vi "Configuration writer.vi"(0 "Path":T1, 1 "Width (px)":i32=240, 2 "error in (no error)":errorcluster, 3 "Precision (%)":dbl=1.0 min=1.0 max=100.0 step=1.0 format="%#_3g", 4 "Heigth (px)":i32=240, 5 "X offset":i32=693 step=1, 6 "X travel":dbl min=0.0 max=50.0 step=0.0001, 7 "Y offset":i32=406 step=1, 10 "Speed (µm/s)":i32=1000, 11 "Height  step \ndivider":i32=2, 12 "Y travel":dbl min=0.0 max=5.0 step=0.0001, 13 "Pixel size":dbl=12.19 step=0.01) -> (19 "error out":errorcluster)   [LabVIEW 2016]
uses:
  <vilib>/Utility/config.llb/Config Data RefNum.ctl
  <vilib>/Utility/config.llb/Write Key (Double).vi
  <vilib>/Utility/config.llb/Write Key (I32).vi
  <vilib>/Utility/config.llb/NI_LVConfig.lvlib
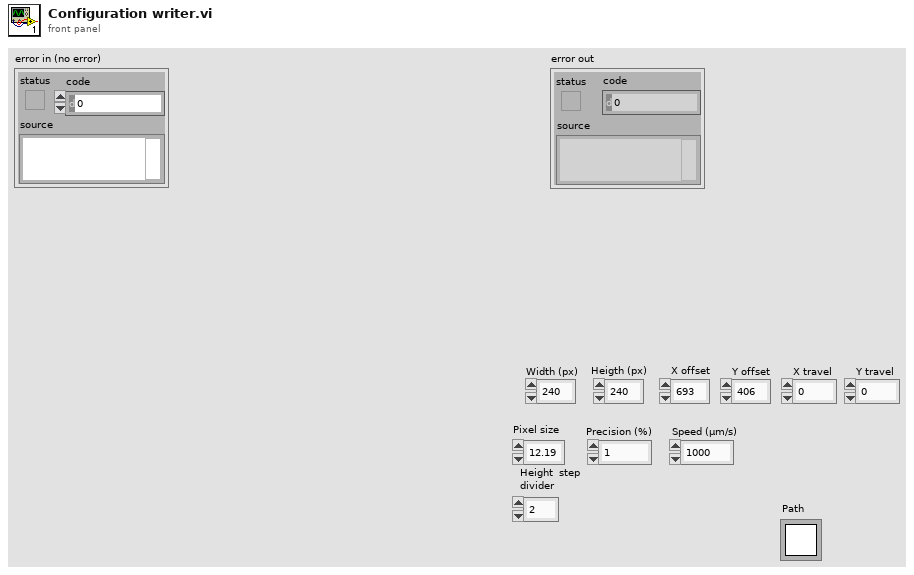
[diagram p1: front panel]
types:
  T1 = typedef "NI_LVConfig.lvlib/Config Data RefNum.ctl" = refnum<k1>
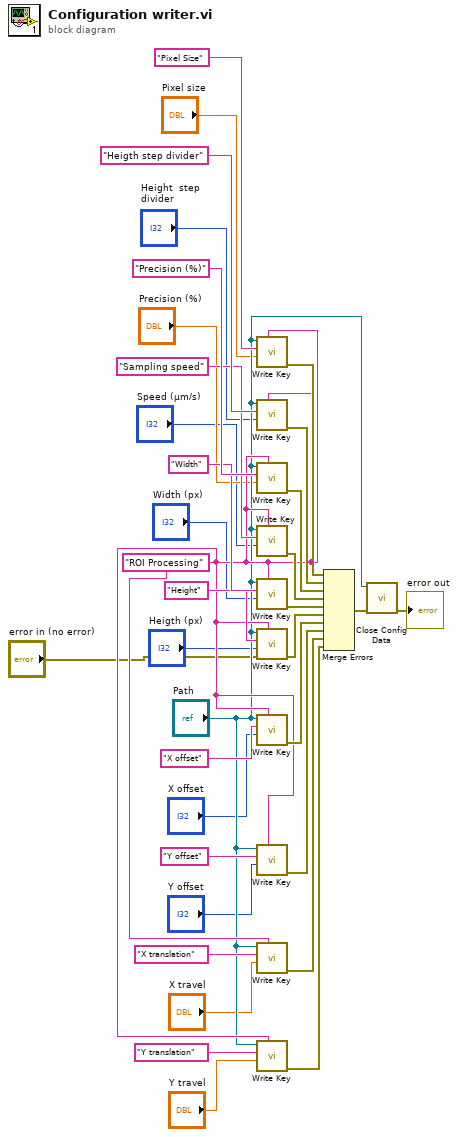
[diagram p0: block diagram]
diagram:
  w18 = "ROI Processing" ("section")
  n1 = call-poly <vilib>:"Write Key.vi"("section"=w18, "value"="Pixel size", "key"="Pixel Size", "refnum"="Path") -> ("error out"=w27:errorcluster)  [unwired: 5 in, 2 out]
  n2 = call-poly <vilib>:"Write Key.vi"("section"=w18, "value"="Height  step \ndivider", "key"="Heigth step divider", "refnum"="Path") -> ("error out"=w26:errorcluster)  [unwired: 5 in, 2 out]
  n3 = call-poly <vilib>:"Write Key.vi"("section"=w18, "value"="Precision (%)", "key"="Precision (%)", "refnum"="Path") -> ("error out"=w25:errorcluster)  [unwired: 5 in, 2 out]
  n4 = call-poly <vilib>:"Write Key.vi"("section"=w18, "value"="Speed (µm/s)", "key"="Sampling speed", "refnum"="Path") -> ("error out"=w24:errorcluster)  [unwired: 5 in, 2 out]
  n5 = call-poly <vilib>:"Write Key.vi"("section"=w18, "value"="Width (px)", "key"="Width", "refnum"="Path") -> ("error out"=w23:errorcluster)  [unwired: 5 in, 2 out]
  n6 = call-poly <vilib>:"Write Key.vi"("section"=w18, "error in (no error)"="error in (no error)", "value"="Heigth (px)", "key"="Height", "refnum"="Path") -> ("error out"=w22:errorcluster)  [unwired: 4 in, 2 out]
  n7 = call-poly <vilib>:"Write Key.vi"("section"=w18, "value"="X offset", "key"="X offset", "refnum"="Path") -> ("error out"=w21:errorcluster)  [unwired: 5 in, 2 out]
  n8 = call-poly <vilib>:"Write Key.vi"("section"=w18, "value"="Y offset", "key"="Y offset", "refnum"="Path") -> ("error out"=w20:errorcluster)  [unwired: 5 in, 2 out]
  n9 = call-poly <vilib>:"Write Key.vi"("section"=w18, "value"="X travel", "key"="X translation", "refnum"="Path") -> ("error out"=w15:errorcluster)  [unwired: 5 in, 2 out]
  n10 = call-poly <vilib>:"Write Key.vi"("section"=w18, "value"="Y travel", "key"="Y translation", "refnum"="Path") -> ("error out"=w14:errorcluster)  [unwired: 5 in, 2 out]
  n11 = Merge Errors(w27, w26, w25, w24, w23, w22, w21, w20, w15, w14) -> (w19:errorcluster)
  n12 = call <vilib>:"Close Config Data.vi"("error in (no error)"=w19, "refnum"="Path") -> ("error out"=→"error out":errorcluster)  [unwired: 8 in, 1 out]
